vi "Picolog Stop Device.vi"(8 "Error In":errorcluster, 11 "Instrument Handle In":i16) -> (0 "Error Out":errorcluster, 3 "Instrument Handle Out":i16)   [LabVIEW 2017]
uses:
  usbtc08.dll
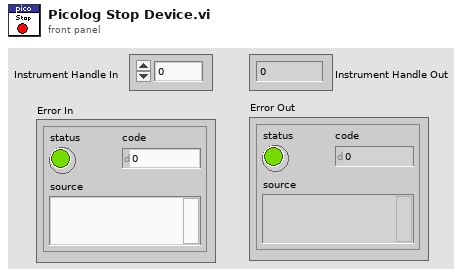
[diagram p1: front panel]
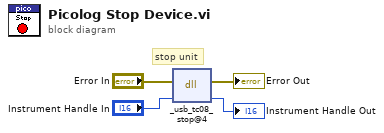
[diagram p0: block diagram]
diagram:
  # "stop unit"
  n1 = dll-call lib="usbtc08.dll" fn="_usb_tc08_stop@4" ("Close unit")(error in="Error In", "handle"="Instrument Handle In") -> (error out=→"Error Out":errorcluster, "handle"=→"Instrument Handle Out":i16)  [unwired: 3 in, 1 out]
